vi "Read Data.vi"(8 "error in (no error)":errorcluster, 11 "Tool Data in":refnum<class "Tool Data.lvclass">) -> (0 "error out":errorcluster, 2 "Data":T1, 3 "Tool Data out":refnum<class "Tool Data.lvclass">)   [LabVIEW 2019, in "Tool Data.lvclass"]
uses:
  Tool Data.lvclass
  Parse/Dot/Dot.lvclass
  Parse/Image/SVGImage.lvclass
  Parse/Rectangle/Rectangle.lvclass
  Parse/ParsePaths/Path.lvclass
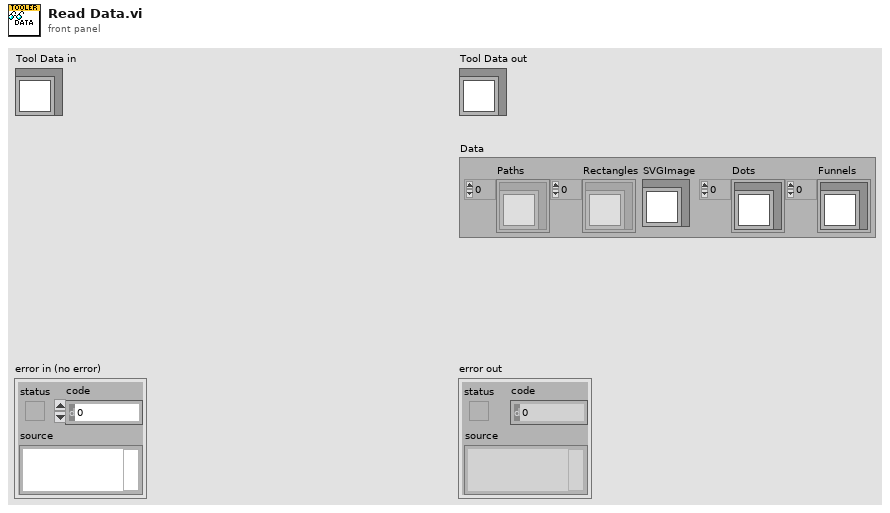
[diagram p1: front panel]
types:
  T1 = cluster{"Paths":refnum<class "Path.lvclass">[], "Rectangles":refnum<class "Rectangle.lvclass">[], "SVGImage":refnum<class "SVGImage.lvclass">, "Dots":refnum<class "Dot.lvclass">[], "Funnels":refnum<class "Path.lvclass">[]}
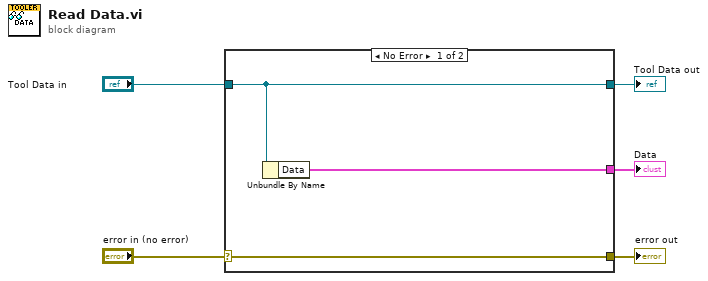
[diagram p0: block diagram]
diagram:
  n1 = case shown="No Error" "error in (no error)" {
    selector: "error in (no error)" -> [w8 w9]
    tunnel: [w8 w9] -> w4
    tunnel: [w7 w10] -> w2
    tunnel: "Tool Data in" -> [w7 w10]
    tunnel: [w6 _] -> w1
    frame No Error {
      n2 = Unbundle By Name(w7) -> ("Data"=w6:T1)
    }
    frame Error {
    }
  }
  "error out" <- w4
  "Tool Data out" <- w2
  "Data" <- w1
